vi "State_Load_Queue.vi"(0 "Immediate actions in":bool[](array[boolean]), 1 "Linked index":i32[](array[numeric]), 2 "Actions":i32[][](array[numeric]), 5 "Current time":timestamp, 7 "Auto actions in":bool[](array[boolean]), 9 "Time of last action":timestamp[](array[timestamp]), 11 "Queue in":i32[](array[numeric]), 12 "Action count in":i32[](array[numeric])) -> (8 "Time til next out":timestamp[](array[timestamp]), 15 "Actions for queue":i32[](array[numeric]))   [LabVIEW 2025]
uses:
  TypeDef_State_Action_Columns.ctl
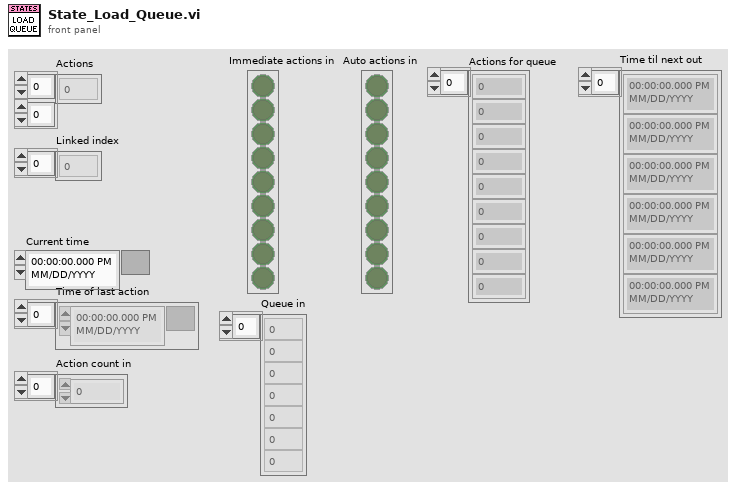
[diagram p1: front panel]
types:
  T1 = typedef "TypeDef_State_Action_Columns.ctl" = enum16{"Action_num", "trigger", "fequency", "offset", "initial state", "mode", "order", "link", "description"}
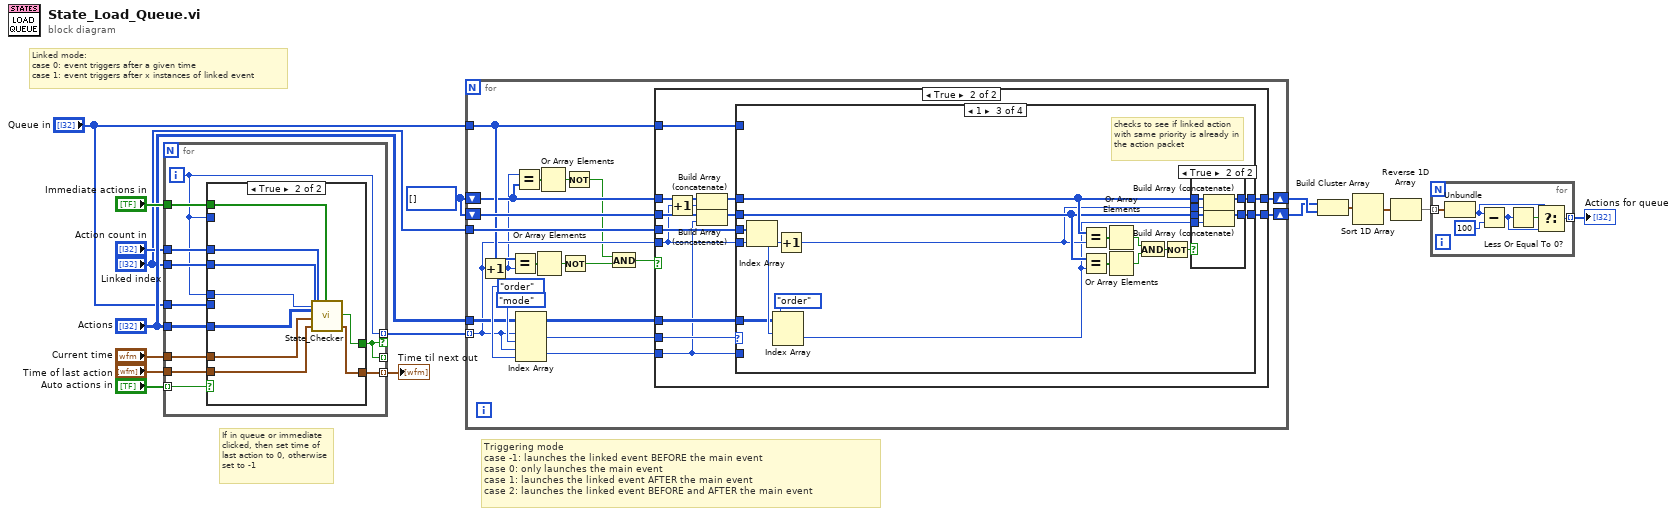
[diagram p0: block diagram]
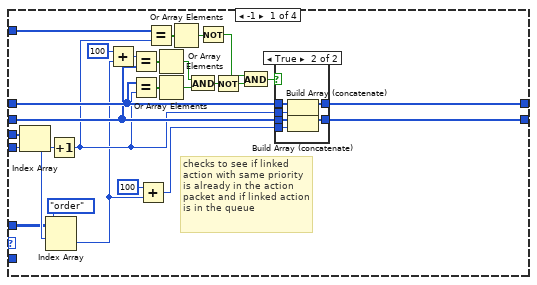
[diagram p3: hidden frame]
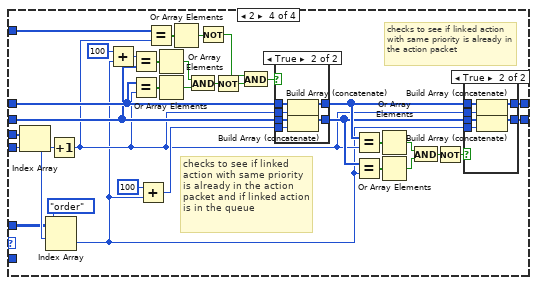
[diagram p7: hidden frame]
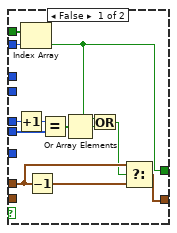
[diagram p10: hidden frame]
diagram:
  w10 = i32[] []
  # "If in queue or immediate clicked, then set time of last action to 0, otherwise set to -1"
  # "Linked mode:\ncase 0: event triggers after a given time\ncase 1: event triggers after x instances of linked event"
  # "Triggering mode\ncase -1: launches the linked event BEFORE the main event\ncase 0: only launches the main event\ncase 1: launches the linked event AFTER the main event\ncase 2: launches the linked event BEFORE and AFTER the main event"
  n1 = for {
    tunnel: "Auto actions in" -> [w25] mode=indexing
    tunnel: "Time of last action" -> [w28]
    tunnel: "Current time" -> [w27]
    tunnel: "Actions" -> [w26]
    tunnel: "Immediate actions in" -> [w24]
    tunnel: [w23] -> _ mode=indexing
    tunnel: [w18] -> w13 mode=indexing if=w23
    tunnel: "Action count in" -> [w22]
    tunnel: "Linked index" -> [w21]
    tunnel: [w20] -> w5 mode=indexing
    tunnel: "Queue in" -> [w19]
    i -> [w18]
    n2 = case shown="True" w25 {
      tunnel: w28 -> [_ w49]
      tunnel: w27 -> [w39 w48]
      tunnel: w26 -> [_ w47]
      tunnel: w24 -> [w31 w43]
      tunnel: [w29 w42] -> w23
      tunnel: w22 -> [_ w46]
      tunnel: w21 -> [_ w45]
      tunnel: [w38 w41] -> w20
      tunnel: w19 -> [w34 _]
      tunnel: w18 -> [w35 w44]
      tunnel: w18 -> [w30 _]
      frame False {
        n3 = Increment(x=w35) -> (x+1=w33:i32)
        n4 = Index Array(array=w31, index=w30) -> (element=w29:bool)
        n5 = Decrement(x=w39) -> (x-1=w40:timestamp)
        n6 = Equal?(x=w33, y=w34) -> (x = y?=w37:bool[])
        n7 = Or Array Elements(Boolean array=w37) -> (logical OR=w32:bool)
        n8 = Or(x=w29, y=w32) -> (x .or. y?=w36:bool)
        n9 = Select(t=w39, s=w36, f=w40) -> (s? t:f=w38:timestamp)
      }
      frame True {
        n10 = call "State_Checker.vi"("Linked index"=w45, "Index"=w44, "Actions"=w47, "Current time"=w48, "Time of last action"=w49, "Action count in"=w46, "Immediate actions in"=w43) -> ("State Ready?"=w42:bool, "Time of next out"=w41:timestamp)  [unwired: 19 in]
      }
    }
  }
  "Time til next out" <- w5
  n11 = for {
    tunnel: w13 -> [w56] mode=indexing
    tunnel: "Actions" -> [w62]
    shift-right: [w66] -> w7
    shift-left: w10 -> [w57]
    shift-right: [w65] -> w6
    shift-left: w10 -> [w67]
    tunnel: "Linked index" -> [w61]
    tunnel: "Queue in" -> [w60]
    n12 = Increment(x=w56) -> (x+1=w52:i32)
    n13 = Equal?(x=w60, y=w52) -> (x = y?=w64:bool[])
    n14 = Equal?(x=w52, y=w57) -> (x = y?=w59:bool[])
    n15 = Index Array(array=w62, index (row) #1=w56, index (col) #1=TypeDef_State_Action_Columns."mode" ("Enum"), index (row) #2=w56, index (col) #2=TypeDef_State_Action_Columns."order" ("Enum")) -> (element #1=w51:i32, element #2=w50:i32)
    n16 = Or Array Elements(Boolean array=w64) -> (logical OR=w63:bool)
    n17 = Or Array Elements(Boolean array=w59) -> (logical OR=w58:bool)
    n18 = Not(x=w63) -> (.not. x?=w54:bool)
    n19 = Not(x=w58) -> (.not. x?=w53:bool)
    n20 = And(x=w53, y=w54) -> (x .and. y?=w55:bool)
    n21 = case shown="True" w55 {
      tunnel: w57 -> [w71 w79]
      tunnel: w67 -> [w70 w78]
      tunnel: [w71 w83] -> w66
      tunnel: [w70 w82] -> w65
      tunnel: w51 -> [_ w84]
      tunnel: w50 -> [_ w75]
      tunnel: w56 -> [_ w73]
      tunnel: w62 -> [_ w81]
      tunnel: w61 -> [_ w80]
      tunnel: w60 -> [_ w74]
      frame False {
      }
      frame True {
        n22 = Increment(x=w73) -> (x+1=w72:i32)
        n23 = Build Array (concatenate)(w79, w72) -> (w77:i32[])
        n24 = Build Array (concatenate)(w78, w75) -> (w76:i32[])
        n25 = case shown="1" w84 {
          tunnel: w77 -> [w90 w120 w124 w153]
          tunnel: w76 -> [w89 w119 w123 w152]
          tunnel: [w110 w120 w137 w179] -> w83
          tunnel: [w109 w119 w136 w178] -> w82
          tunnel: w75 -> [_ _ _ _]
          tunnel: w73 -> [w106 _ w128 w170]
          tunnel: w81 -> [w104 _ w126 w168]
          tunnel: w80 -> [w105 _ w127 w169]
          tunnel: w74 -> [w102 _ _ w165]
          frame -1 {
            # "checks to see if linked action with same priority is already in the action packet and if linked action is in the queue"
            n26 = Index Array(array=w105, index=w106) -> (element=w107:i32)
            n27 = Index Array(array=w104, index (row)=w107, index (col)=TypeDef_State_Action_Columns."order" ("Enum")) -> (element=w85:i32)
            n28 = Increment(x=w107) -> (x+1=w86:i32)
            n29 = Add(x=100, y=w85) -> (x+y=w94:i32)
            n30 = Equal?(x=w94, y=w89) -> (x = y?=w100:bool[])
            n31 = Equal?(x=w90, y=w86) -> (x = y?=w99:bool[])
            n32 = Add(x=100, y=w85) -> (x+y=w87:i32)
            n33 = Equal?(x=w102, y=w86) -> (x = y?=w103:bool[])
            n34 = Or Array Elements(Boolean array=w100) -> (logical OR=w98:bool)
            n35 = Or Array Elements(Boolean array=w99) -> (logical OR=w97:bool)
            n36 = Or Array Elements(Boolean array=w103) -> (logical OR=w101:bool)
            n37 = And(x=w98, y=w97) -> (x .and. y?=w96:bool)
            n38 = Not(x=w101) -> (.not. x?=w93:bool)
            n39 = Not(x=w96) -> (.not. x?=w92:bool)
            n40 = And(x=w93, y=w92) -> (x .and. y?=w91:bool)
            n41 = case shown="True" w91 {
              tunnel: w90 -> [w112 w118]
              tunnel: [w112 w116] -> w110
              tunnel: w89 -> [w111 w117]
              tunnel: [w111 w115] -> w109
              tunnel: w87 -> [_ w114]
              tunnel: w86 -> [_ w113]
              frame False {
              }
              frame True {
                n42 = Build Array (concatenate)(w118, w113) -> (w116:i32[])
                n43 = Build Array (concatenate)(w117, w114) -> (w115:i32[])
              }
            }
          }
          frame 0, Default {
            # "no linked action, so once main event is added, don't need to do anything else"
          }
          frame 1 {
            # "checks to see if linked action with same priority is already in the action packet"
            n44 = Index Array(array=w127, index=w128) -> (element=w132:i32)
            n45 = Index Array(array=w126, index (row)=w132, index (col)=TypeDef_State_Action_Columns."order" ("Enum")) -> (element=w121:i32)
            n46 = Increment(x=w132) -> (x+1=w122:i32)
            n47 = Equal?(x=w124, y=w122) -> (x = y?=w135:bool[])
            n48 = Equal?(x=w123, y=w121) -> (x = y?=w134:bool[])
            n49 = Or Array Elements(Boolean array=w135) -> (logical OR=w131:bool)
            n50 = Or Array Elements(Boolean array=w134) -> (logical OR=w130:bool)
            n51 = And(x=w131, y=w130) -> (x .and. y?=w129:bool)
            n52 = Not(x=w129) -> (.not. x?=w125:bool)
            n53 = case shown="True" w125 {
              tunnel: w124 -> [w139 w145]
              tunnel: [w139 w143] -> w137
              tunnel: w123 -> [w138 w144]
              tunnel: [w138 w142] -> w136
              tunnel: w121 -> [_ w141]
              tunnel: w122 -> [_ w140]
              frame False {
              }
              frame True {
                n54 = Build Array (concatenate)(w145, w140) -> (w143:i32[])
                n55 = Build Array (concatenate)(w144, w141) -> (w142:i32[])
              }
            }
          }
          frame 2 {
            # "checks to see if linked action with same priority is already in the action packet and if linked action is in the queue"
            # "checks to see if linked action with same priority is already in the action packet"
            n56 = Index Array(array=w169, index=w170) -> (element=w174:i32)
            n57 = Index Array(array=w168, index (row)=w174, index (col)=TypeDef_State_Action_Columns."order" ("Enum")) -> (element=w146:i32)
            n58 = Increment(x=w174) -> (x+1=w147:i32)
            n59 = Add(x=100, y=w146) -> (x+y=w157:i32)
            n60 = Equal?(x=w157, y=w152) -> (x = y?=w163:bool[])
            n61 = Equal?(x=w153, y=w147) -> (x = y?=w162:bool[])
            n62 = Add(x=100, y=w146) -> (x+y=w148:i32)
            n63 = Equal?(x=w165, y=w147) -> (x = y?=w166:bool[])
            n64 = Or Array Elements(Boolean array=w163) -> (logical OR=w161:bool)
            n65 = Or Array Elements(Boolean array=w162) -> (logical OR=w160:bool)
            n66 = Or Array Elements(Boolean array=w166) -> (logical OR=w164:bool)
            n67 = And(x=w161, y=w160) -> (x .and. y?=w159:bool)
            n68 = Not(x=w164) -> (.not. x?=w156:bool)
            n69 = Not(x=w159) -> (.not. x?=w155:bool)
            n70 = And(x=w156, y=w155) -> (x .and. y?=w154:bool)
            n71 = case shown="True" w154 {
              tunnel: w153 -> [w181 w187]
              tunnel: [w181 w185] -> w151
              tunnel: w152 -> [w180 w186]
              tunnel: [w180 w184] -> w150
              tunnel: w148 -> [_ w183]
              tunnel: w147 -> [_ w182]
              frame False {
              }
              frame True {
                n72 = Build Array (concatenate)(w187, w182) -> (w185:i32[])
                n73 = Build Array (concatenate)(w186, w183) -> (w184:i32[])
              }
            }
            n74 = Equal?(x=w151, y=w147) -> (x = y?=w177:bool[])
            n75 = Equal?(x=w150, y=w146) -> (x = y?=w176:bool[])
            n76 = Or Array Elements(Boolean array=w177) -> (logical OR=w173:bool)
            n77 = Or Array Elements(Boolean array=w176) -> (logical OR=w172:bool)
            n78 = And(x=w173, y=w172) -> (x .and. y?=w171:bool)
            n79 = Not(x=w171) -> (.not. x?=w167:bool)
            n80 = case shown="True" w167 {
              tunnel: w151 -> [w189 w195]
              tunnel: [w189 w193] -> w179
              tunnel: w150 -> [w188 w194]
              tunnel: [w188 w192] -> w178
              tunnel: w146 -> [_ w191]
              tunnel: w147 -> [_ w190]
              frame False {
              }
              frame True {
                n81 = Build Array (concatenate)(w195, w190) -> (w193:i32[])
                n82 = Build Array (concatenate)(w194, w191) -> (w192:i32[])
              }
            }
          }
        }
      }
    }
  }
  n83 = Build Cluster Array(w6, w7) -> (w8:cluster{i32, i32}[])
  n84 = Sort 1D Array(array=w8) -> (sorted array=w3:cluster{i32, i32}[])
  n85 = Reverse 1D Array(array=w3) -> (reversed array=w2:cluster{i32, i32}[])
  n86 = for {
    tunnel: w2 -> [w201] mode=indexing
    tunnel: [w196] -> w1 mode=indexing
    n87 = Unbundle(w201) -> (w198:i32)  [unwired: 1 out]
    n88 = Subtract(x=w198, y=100) -> (x-y=w197:i32)
    n89 = Less Or Equal To 0?(x=w197) -> (x <= 0?=w199:bool)
    n90 = Select(t=w198, s=w199, f=w197) -> (s? t:f=w196:i32)
  }
  "Actions for queue" <- w1
